vi "ValveGUI.vi"() -> ()   [LabVIEW 2020, in "VolatusScratch.lvlib"]
uses:
  VolatusScratch.lvlib
  VolatusGUIControls/2WayValveH.ctl
  VolatusGUIControls/DblNumericStatus.ctl
  VolatusGUIControls/DblControl.ctl
  VolatusGUIControls/ButtonControl.ctl
  VolatusGUIControls/Logging Control.ctl
  VolatusGUIControls/VolatusGUIControls.lvlib
panel:
  in  "Logging Control":T1
  in  "PulseBtn":T2
  in  "Unpulsed":T3={"Picture"=bytes[9690], "Command"=FALSE}
  in  "AO 0":T4
  in  "Seq1 Delay s":T4
  in  "Pulse2 s":T4
  in  "Pulse1 s":T4
  in  "Seq1":T3={"Picture"=bytes[9690], "Command"=FALSE}
  in  "Pulse2":T3={"Picture"=bytes[9690], "Command"=FALSE}
  in  "Pulse1":T3={"Picture"=bytes[9690], "Command"=FALSE}
  out "AI 1":T5
  out "AI 0":T5
  out "Latch1":T5
  in  "Latch1":T3={"Picture"=bytes[9690], "Command"=FALSE}
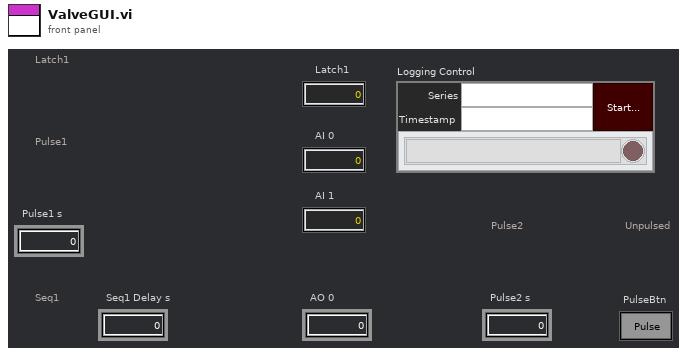
[diagram p1: front panel]
types:
  T1 = typedef "VolatusGUIControls.lvlib/Logging Control.ctl" = cluster{"Series":string, "Timestamp":string, "Log Button":bool, "Status":cluster{"Node":string, "Logging":bool}[]}
  T2 = typedef "VolatusGUIControls.lvlib/ButtonControl.ctl" = cluster{"Color":u32, "Button":bool}
  T3 = typedef "VolatusGUIControls.lvlib/2WayValveH.ctl" = cluster{"Picture":picture, "Command":bool}
  T4 = typedef "VolatusGUIControls.lvlib/DblControl.ctl" = cluster{"Color":u32, "Value":dbl, "Backdrop":bool}
  T5 = typedef "VolatusGUIControls.lvlib/DblNumericStatus.ctl" = cluster{"Color":u32, "Value":dbl}
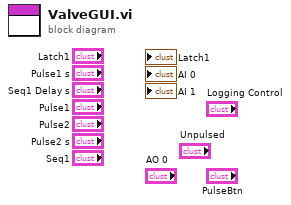
[diagram p0: block diagram]
diagram:
